vi "Test Parse Error Snippet.vi"(8 "error in (no error)":errorcluster) -> (0 "error out":errorcluster)   [LabVIEW 2020]
uses:
  src/Deserializer/JSON Deserializer/JSON Deserializer.lvclass
  <vilib>/addons/_JKI Toolkits/Caraya/classes/Assert/Assert True.vi
  <vilib>/addons/_JKI Toolkits/Caraya/classes/Test/Test.lvclass
  <vilib>/addons/_JKI Toolkits/Caraya/classes/Assert/Assert.lvclass
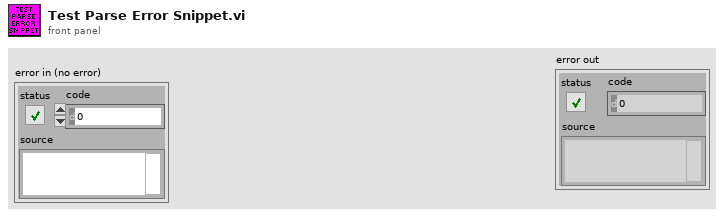
[diagram p1: front panel]
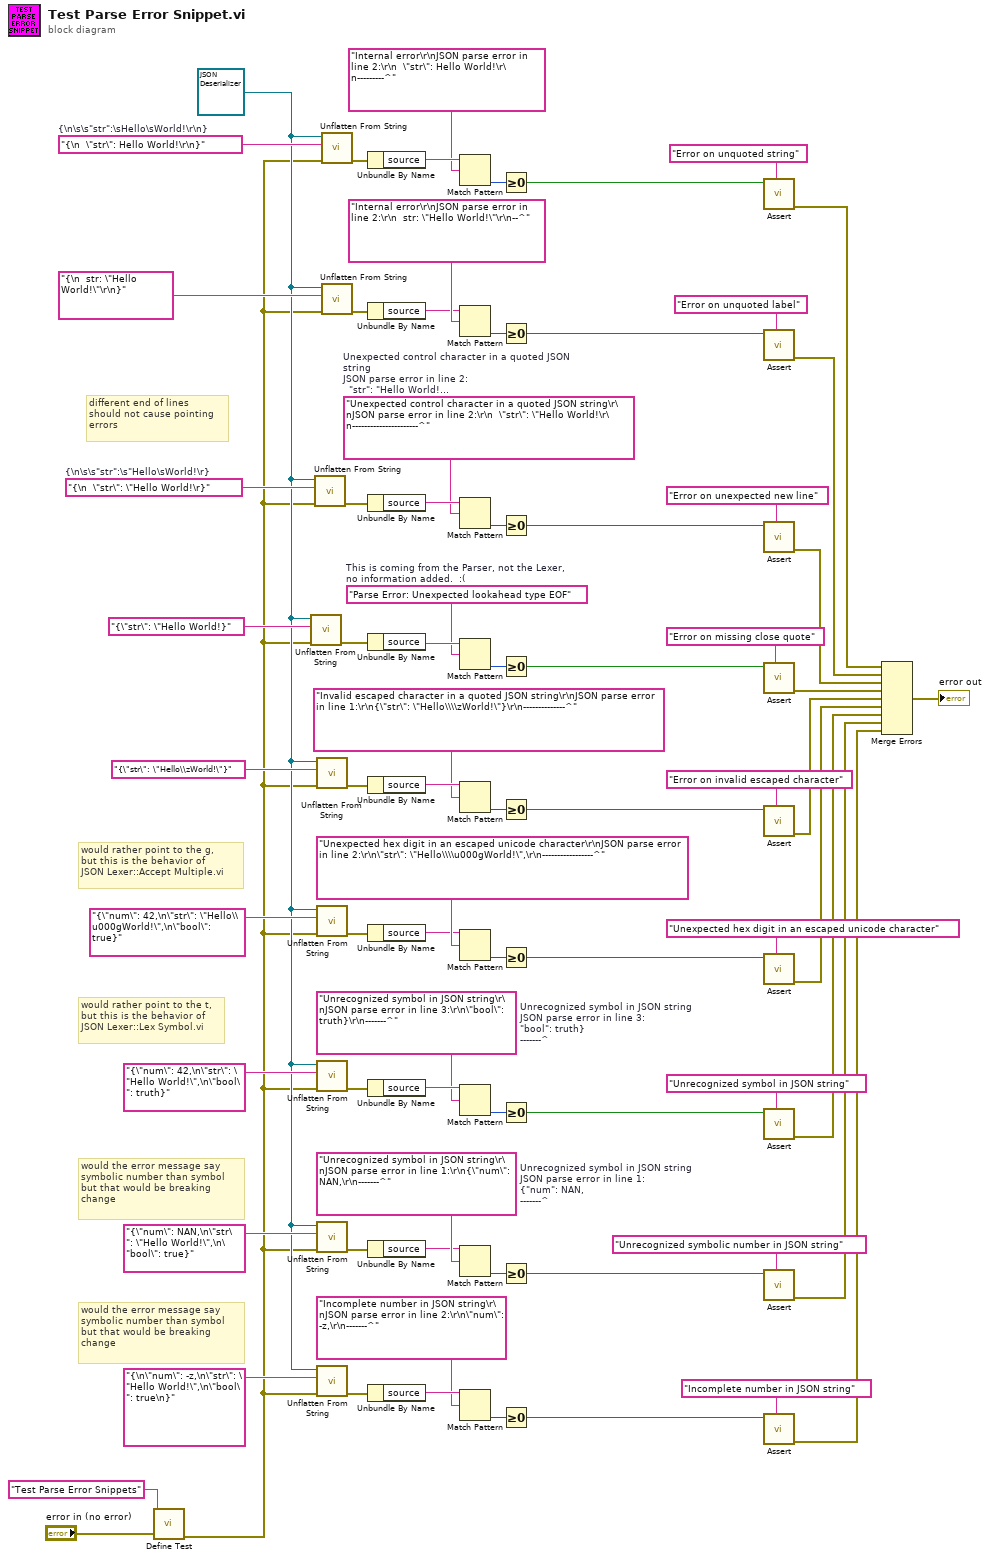
[diagram p0: block diagram]
diagram:
  w25 = "Unrecognized symbol in JSON string\r\nJSON parse error in line 1:\r\n{\"num\": NAN,\r\n-------^"  # Unrecognized symbol in JSON string JSON parse error in line 1: {"num": NAN, -------^
  w29 = "Unrecognized symbol in JSON string\r\nJSON parse error in line 3:\r\n\"bool\": truth}\r\n-------^"  # Unrecognized symbol in JSON string JSON parse error in line 3: "bool": truth} -------^
  w51 = "Parse Error: Unexpected lookahead type EOF"  # This is coming from the Parser, not the Lexer, no information added.  :(
  w57 = "{\n  \"str\": \"Hello World!\r}"  # {\n\s\s"str":\s"Hello\sWorld!\r}
  w58 = "Unexpected control character in a quoted JSON string\r\nJSON parse error in line 2:\r\n  \"str\": \"Hello World!\r\n----------------------^"  # Unexpected control character in a quoted JSON string JSON parse error in line 2:   "str": "Hello World! ----------------------^
  w3 = refnum<class "JSON Deserializer.lvclass"> refnum ("Deserializer in")
  w70 = "{\n  \"str\": Hello World!\r\n}"  # {\n\s\s"str":\sHello\sWorld!\r\n}
  # "would the error message say\nsymbolic number than symbol\nbut that would be breaking\nchange"
  # "would the error message say\nsymbolic number than symbol\nbut that would be breaking\nchange"
  # "would rather point to the t,\nbut this is the behavior of\nJSON Lexer::Lex Symbol.vi"
  # "would rather point to the g,\nbut this is the behavior of\nJSON Lexer::Accept Multiple.vi"
  # "different end of lines\nshould not cause pointing\nerrors"
  n1 = call <vilib>:"Define Test.vi"("error in (no error)"="error in (no error)", "Label (VI Title)"="Test Parse Error Snippets") -> ("error out"=w2:errorcluster)  [unwired: 8 in, 1 out]
  n2 = call-dynamic "Unflatten From String.vi"("error in (no error)"=w2, "String"="{\"str\": \"Hello World!}", "Deserializer in"=w3) -> ("error out"=w72:errorcluster)  [unwired: 6 in, 2 out]
  n3 = call-dynamic "Unflatten From String.vi"("error in (no error)"=w2, "String"=w57, "Deserializer in"=w3) -> ("error out"=w73:errorcluster)  [unwired: 6 in, 2 out]
  n4 = call-dynamic "Unflatten From String.vi"("error in (no error)"=w2, "String"="{\"str\": \"Hello\\zWorld!\"}", "Deserializer in"=w3) -> ("error out"=w71:errorcluster)  [unwired: 6 in, 2 out]
  n5 = call-dynamic "Unflatten From String.vi"("error in (no error)"=w2, "String"="{\"num\": 42,\n\"str\": \"Hello\\u000gWorld!\",\n\"bool\": true}", "Deserializer in"=w3) -> ("error out"=w36:errorcluster)  [unwired: 6 in, 2 out]
  n6 = call-dynamic "Unflatten From String.vi"("error in (no error)"=w2, "String"="{\"num\": 42,\n\"str\": \"Hello World!\",\n\"bool\": truth}", "Deserializer in"=w3) -> ("error out"=w34:errorcluster)  [unwired: 6 in, 2 out]
  n7 = call-dynamic "Unflatten From String.vi"("error in (no error)"=w2, "String"="{\"num\": NAN,\n\"str\": \"Hello World!\",\n\"bool\": true}", "Deserializer in"=w3) -> ("error out"=w21:errorcluster)  [unwired: 6 in, 2 out]
  n8 = call-dynamic "Unflatten From String.vi"("error in (no error)"=w2, "String"="{\n\"num\": -z,\n\"str\": \"Hello World!\",\n\"bool\": true\n}", "Deserializer in"=w3) -> ("error out"=w18:errorcluster)  [unwired: 6 in, 2 out]
  n9 = call-dynamic "Unflatten From String.vi"("error in (no error)"=w2, "String"=w70, "Deserializer in"=w3) -> ("error out"=w74:errorcluster)  [unwired: 6 in, 2 out]
  n10 = call-dynamic "Unflatten From String.vi"("error in (no error)"=w2, "String"="{\n  str: \"Hello World!\"\r\n}", "Deserializer in"=w3) -> ("error out"=w5:errorcluster)  [unwired: 6 in, 2 out]
  n11 = Unbundle By Name(w74) -> ("source"=w64:string)
  n12 = Unbundle By Name(w5) -> ("source"=w9:string)
  n13 = Unbundle By Name(w73) -> ("source"=w60:string)
  n14 = Unbundle By Name(w72) -> ("source"=w53:string)
  n15 = Unbundle By Name(w71) -> ("source"=w45:string)
  n16 = Unbundle By Name(w36) -> ("source"=w40:string)
  n17 = Unbundle By Name(w34) -> ("source"=w30:string)
  n18 = Unbundle By Name(w21) -> ("source"=w24:string)
  n19 = Unbundle By Name(w18) -> ("source"=w15:string)
  n20 = Match Pattern(string=w64, regular expression="Internal error\r\nJSON parse error in line 2:\r\n  \"str\": Hello World!\r\n---------^") -> (offset past match=w69:i32)  [unwired: 1 in, 3 out]
  n21 = Match Pattern(string=w9, regular expression="Internal error\r\nJSON parse error in line 2:\r\n  str: \"Hello World!\"\r\n--^") -> (offset past match=w7:i32)  [unwired: 1 in, 3 out]
  n22 = Match Pattern(string=w60, regular expression=w58) -> (offset past match=w61:i32)  [unwired: 1 in, 3 out]
  n23 = Match Pattern(string=w53, regular expression=w51) -> (offset past match=w55:i32)  [unwired: 1 in, 3 out]
  n24 = Match Pattern(string=w45, regular expression="Invalid escaped character in a quoted JSON string\r\nJSON parse error in line 1:\r\n{\"str\": \"Hello\\\\zWorld!\"}\r\n--------------^") -> (offset past match=w47:i32)  [unwired: 1 in, 3 out]
  n25 = Match Pattern(string=w40, regular expression="Unexpected hex digit in an escaped unicode character\r\nJSON parse error in line 2:\r\n\"str\": \"Hello\\\\u000gWorld!\",\r\n-----------------^") -> (offset past match=w39:i32)  [unwired: 1 in, 3 out]
  n26 = Match Pattern(string=w30, regular expression=w29) -> (offset past match=w31:i32)  [unwired: 1 in, 3 out]
  n27 = Match Pattern(string=w24, regular expression=w25) -> (offset past match=w23:i32)  [unwired: 1 in, 3 out]
  n28 = Match Pattern(string=w15, regular expression="Incomplete number in JSON string\r\nJSON parse error in line 2:\r\n\"num\": -z,\r\n-------^") -> (offset past match=w16:i32)  [unwired: 1 in, 3 out]
  n29 = Greater Or Equal To 0?(x=w69) -> (x >= 0?=w68:bool)
  n30 = Greater Or Equal To 0?(x=w7) -> (x >= 0?=w8:bool)
  n31 = Greater Or Equal To 0?(x=w61) -> (x >= 0?=w62:bool)
  n32 = Greater Or Equal To 0?(x=w55) -> (x >= 0?=w52:bool)
  n33 = Greater Or Equal To 0?(x=w47) -> (x >= 0?=w49:bool)
  n34 = Greater Or Equal To 0?(x=w39) -> (x >= 0?=w37:bool)
  n35 = Greater Or Equal To 0?(x=w31) -> (x >= 0?=w33:bool)
  n36 = Greater Or Equal To 0?(x=w23) -> (x >= 0?=w22:bool)
  n37 = Greater Or Equal To 0?(x=w16) -> (x >= 0?=w17:bool)
  n38 = call-poly <vilib>:"Assert.vi"("Label"="Error on unquoted string", "True?"=w68) -> ("error out"=w66:errorcluster)  [unwired: 8 in, 1 out]
  n39 = call-poly <vilib>:"Assert.vi"("Label"="Error on unquoted label", "True?"=w8) -> ("error out"=w1:errorcluster)  [unwired: 8 in, 1 out]
  n40 = call-poly <vilib>:"Assert.vi"("Label"="Error on unexpected new line", "True?"=w62) -> ("error out"=w56:errorcluster)  [unwired: 8 in, 1 out]
  n41 = call-poly <vilib>:"Assert.vi"("Label"="Error on missing close quote", "True?"=w52) -> ("error out"=w50:errorcluster)  [unwired: 8 in, 1 out]
  n42 = call-poly <vilib>:"Assert.vi"("Label"="Error on invalid escaped character", "True?"=w49) -> ("error out"=w46:errorcluster)  [unwired: 8 in, 1 out]
  n43 = call-poly <vilib>:"Assert.vi"("Label"="Unexpected hex digit in an escaped unicode character", "True?"=w37) -> ("error out"=w35:errorcluster)  [unwired: 8 in, 1 out]
  n44 = call-poly <vilib>:"Assert.vi"("Label"="Unrecognized symbol in JSON string", "True?"=w33) -> ("error out"=w27:errorcluster)  [unwired: 8 in, 1 out]
  n45 = call-poly <vilib>:"Assert.vi"("Label"="Unrecognized symbolic number in JSON string", "True?"=w22) -> ("error out"=w19:errorcluster)  [unwired: 8 in, 1 out]
  n46 = call-poly <vilib>:"Assert.vi"("Label"="Incomplete number in JSON string", "True?"=w17) -> ("error out"=w11:errorcluster)  [unwired: 8 in, 1 out]
  n47 = Merge Errors(w66, w1, w56, w50, w46, w35, w27, w19, w11) -> (→"error out":errorcluster)
